vi "stack-temp-tuner.vi"() -> ()   [LabVIEW 2019]
uses:
  <vilib>/Analysis/NI_AALPro.lvlib
panel:
  in  "hyst":sgl=25.0
  in  "boost":sgl=25.0
  in  "boost_delay":u8=25
  in  "Alarm State":bool=TRUE
  in  "Alarm Enable":bool=TRUE
  in  "Mute":bool
  in  "Mute Time (min)":u8=1
  in  "Alarm Diff":u8=30
  in  "Write Manual Coeffs":bool
  in  "Manual Coeffs":sgl[](array[numeric])=[0.0, 1.0]
  in  "Live Data":bool=TRUE
  out "Version":sgl format="%#.1f"
  in  "System Type":u8(ring) items=["Stack Temp", "Auto Draw-Off"]
  in  "pwm_min":u8=25
  in  "ff":sgl
  in  "Output Enable Type":bool
  out "Cal Read 2":sgl format="%#.1g"
  out "Cal Read 1":sgl
  in  "Cal Target 2":sgl=900.0 min=32 max=2000 step=1
  in  "Cal Target 1":sgl=32.0 min=32 max=2000 step=1
  in  "Apply Cal":bool
  out "Temp (deg F)":sgl=78.2392 format="%.1f"
  out "Temp (raw)":sgl=554.0 format="%#.1f"
  in  "Cal Capture 2":bool
  in  "Cal Capture 1":bool
  in  "Received Reset":bool
  out "Parameters Received":bool
  out "Cal Coeffs":sgl[](array[numeric])
  in  "Parameter Request":bool
  in  "Output Enable":bool=TRUE
  in  "pwm_rate":sgl=50.0
  in  "ki":sgl=0.001
  in  "kp":sgl=5.0
  in  "Write Tuning":bool
  in  "Temp Setpoint":sgl=100.0 min=32 max=1832 step=0.1 format="%#.1f"
  out "Live Data":sgl[](array[numeric])=[78.2392, 100.0, 118.0, 9295.232] format="%.1f"
  out "Tuning Chart":T1(graph)={"[0]"=78.2392, "[1]"=100.0, "[2]"=118.0, "[3]"=9295.232, "[4]"=0.0, "[5]"=0.0, "[6]"=0.0, "[7]"=0.0, "[8]"=0.0}
  in  "Stop":bool
  # "Control"
  # "Parameter Request"
  # "Config"
  # "Tuning"
  # "Temp Calibration"
  # "Manual Coeffs"
  # "Stack Temp Alarm"
  # "*Any kp over 5 will cause the command\nstep to increase from 1 to 2.  This is due to\nthe resolution of the temp input (at least\nfor stack temp anyway)"
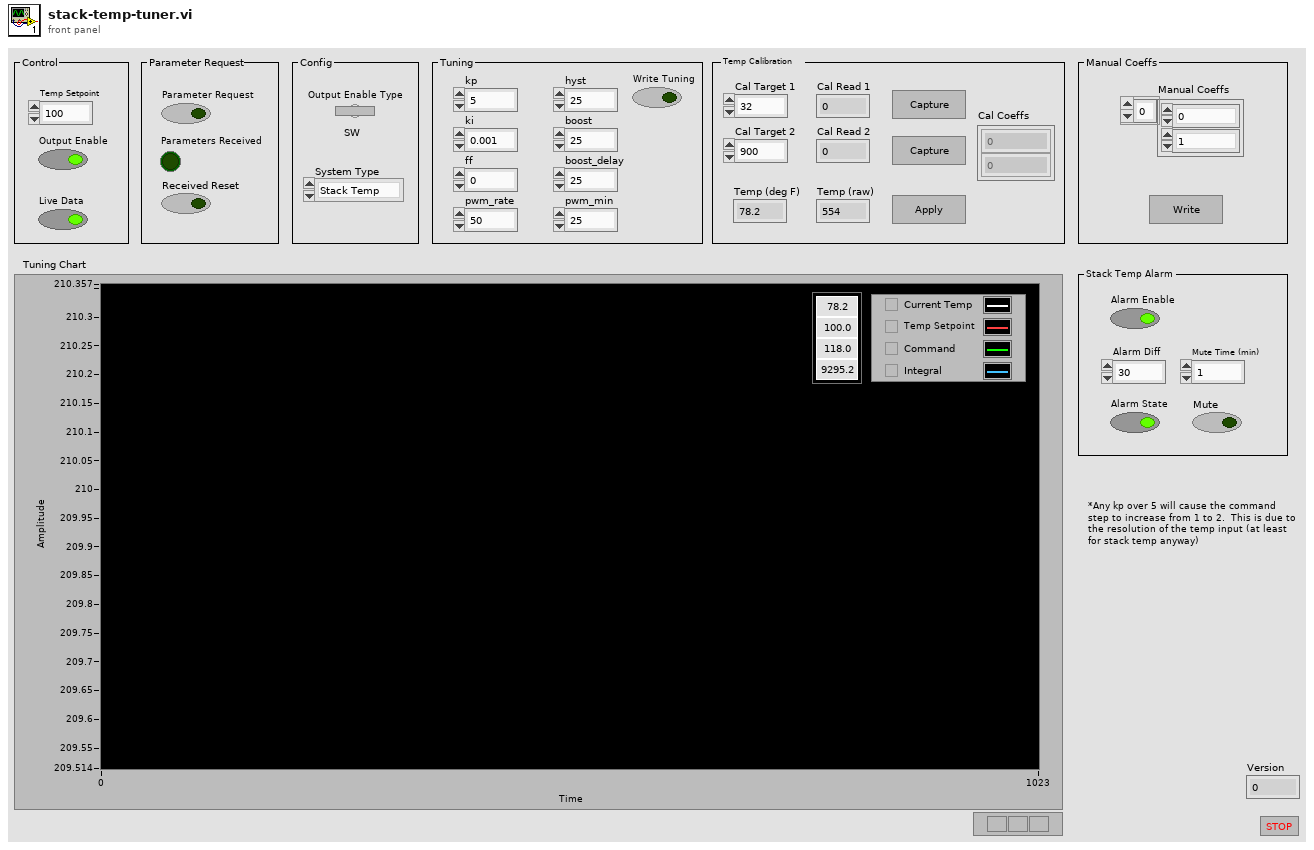
[diagram p1: front panel]
types:
  T1 = cluster{"[0]":sgl, "[1]":sgl, "[2]":sgl, "[3]":sgl, "[4]":sgl, "[5]":sgl, "[6]":sgl, "[7]":sgl, "[8]":sgl}
  T2 = cluster{"Error":errorcluster, "CAN Object":i32, "CAN Msg":u8[], "ArbID":u32, "Cal Coeffs":sgl[], "Current Temp":sgl, "Temp (raw)":sgl, "Temp Setpoint":sgl, "Output Enable":bool, "Parameter Request":bool, "Parameter Received":bool, "Cal Target 1":sgl, "Cal Target 2":sgl, "Cal Read 1":sgl, "Cal Read 2":sgl, "kp":sgl, "ki":sgl, "pwm_rate":sgl, "ff":sgl, "hyst":sgl, "boost":sgl, "pwm_min":u8, "boost_delay":u8, "Temp Setpoint (Live)":sgl, "Integral":sgl, "PWM Command":sgl, "Output Enable Type":bool, "System Type":u8, "Version":sgl, "Alarm Diff":u8, "Alarm Enable":bool, "Mute Time (min)":u8, "Alarm State":bool}
  T3 = enum16{"DEVICE", "HSCAN", "MSCAN", "SWCAN", "LSFTCAN", "FORDSCP", "J1708", "JVPW", "ISO", "FIRE_HSCAN2", "FIRE_MSCAN1", "FIRE_HSCAN3", "FIRE_LIN2", "FIRE_LIN3", "FIRE_LIN4"}
  T4 = cluster{"DeviceType":i32, "Handle":i32, "NumberOfClients":i32, "SerialNumber":i32, "MaxAllowedClients":i32}[]
  T5 = cluster{"DeviceType":i32, "Handle":i32, "NumberOfClients":i32, "SerialNumber":i32, "MaxAllowedClients":i32}
  T6 = typedef "ctl spymessage.ctl" = cluster{"StatusBitField":u32, "StatusBitField2":u32, "TimeHardware":u32, "TimeHardware2":u32, "TimeSystem":u32, "TimeSystem2":u32, "TimeStampHardwareID":u8, "TimeStampHardwareID2":u8, "NetworkID":u8, "NodeID":u8, "Protocol":u8, "MessagePieceID":u8, "ColorID":u8, "NumberBytesHeader":u8, "NumberBytesData":u8, "DescriptionID":u16, "ArbIDOrHeader":u32, "Data [8]":u8[], "AckBytes [8]":u8[], "Value":sgl, "MiscData":u8}
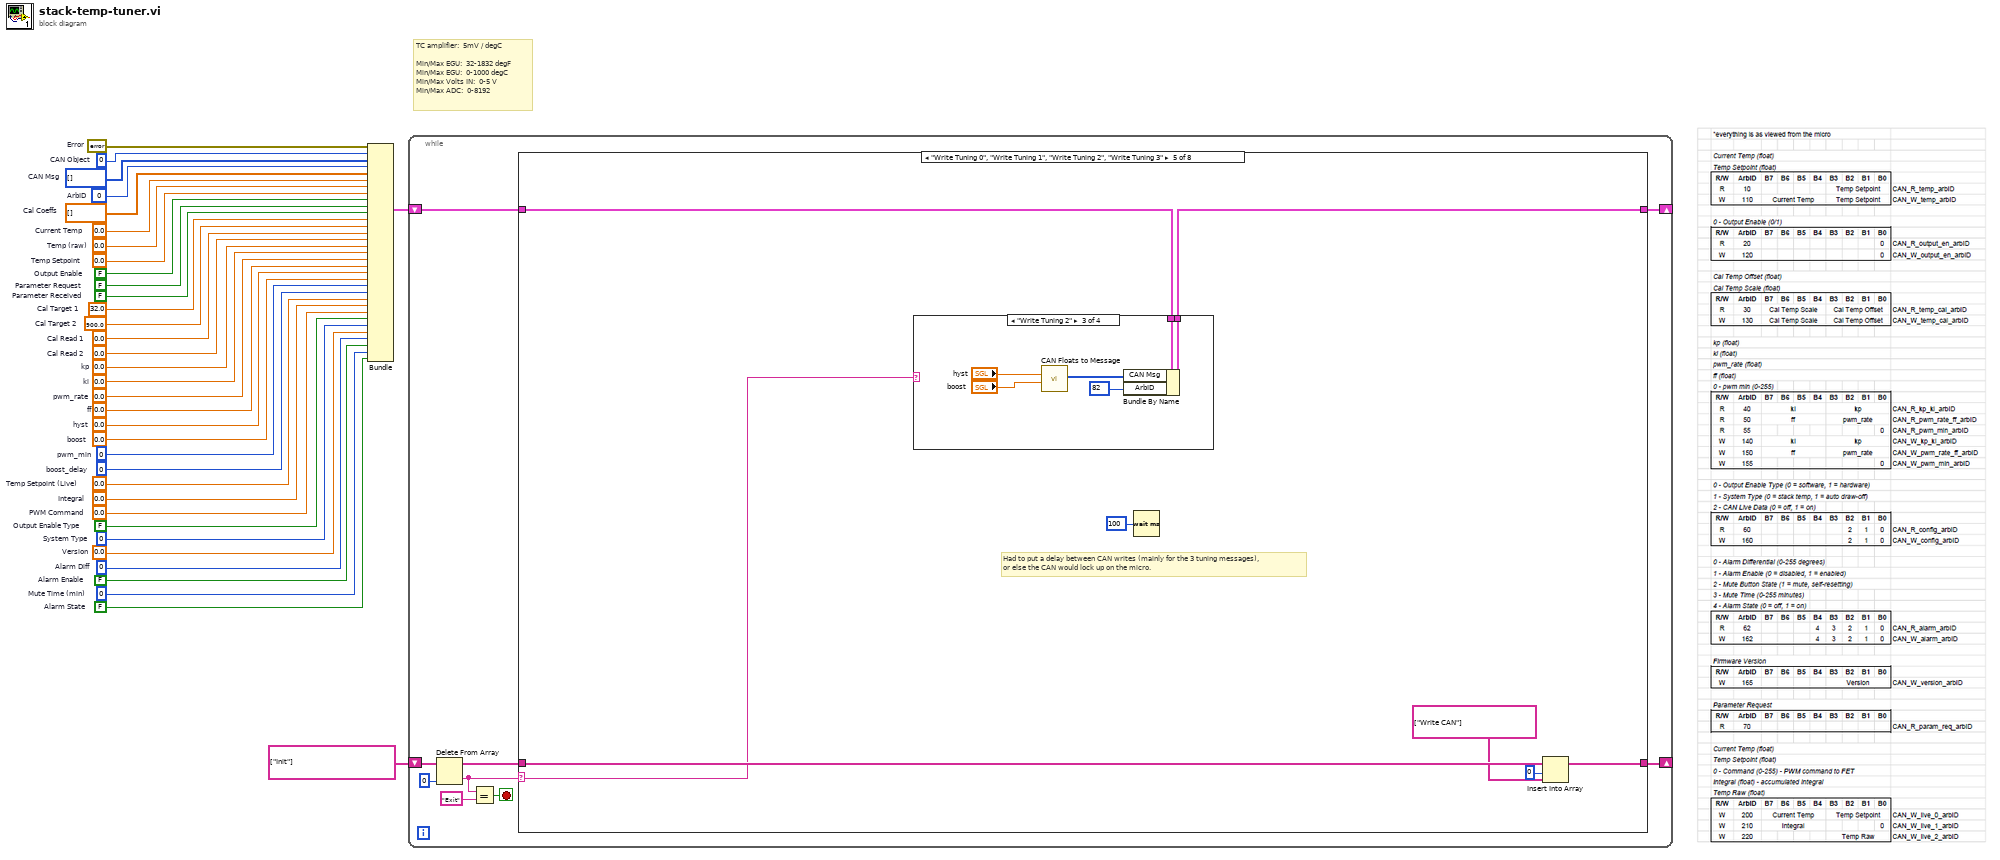
[diagram p0: block diagram]
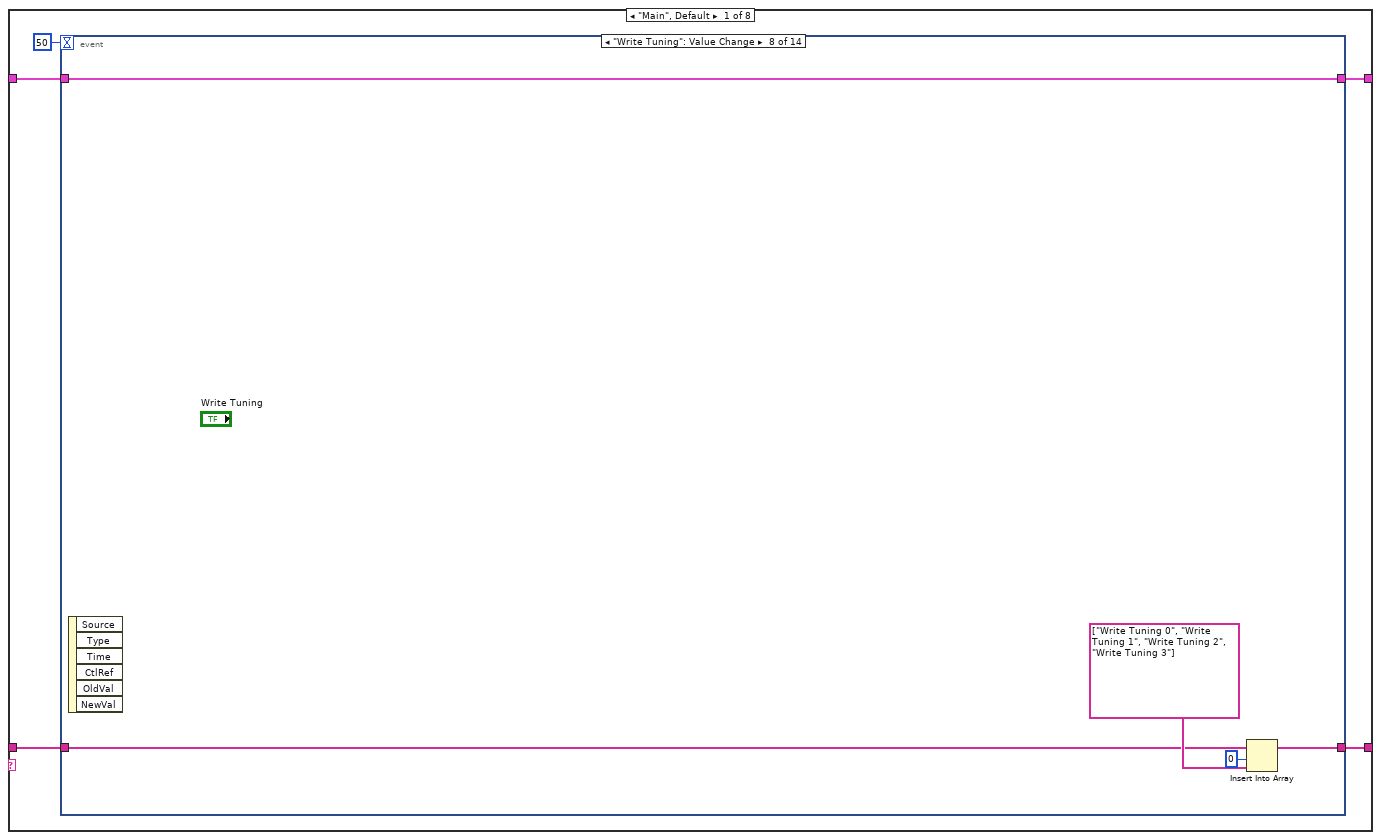
[diagram p2: hidden frame]
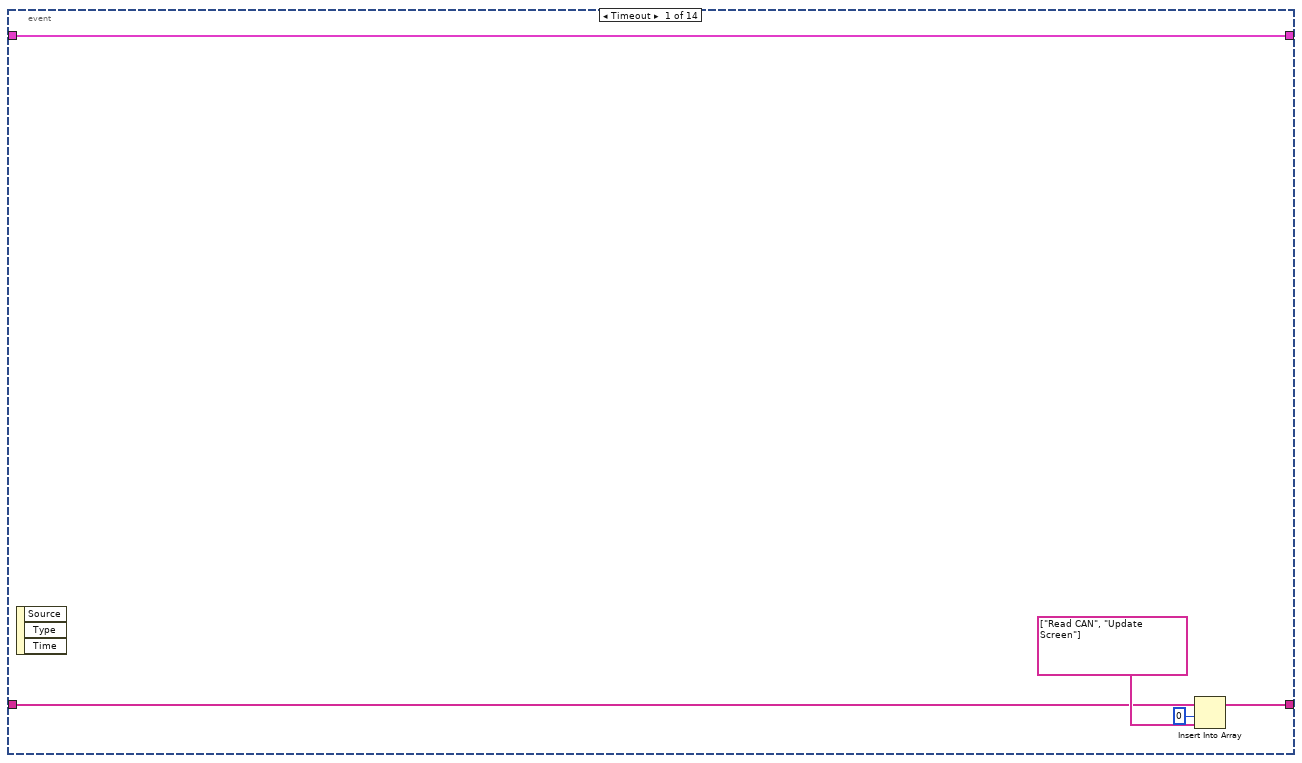
[diagram p3: hidden frame]
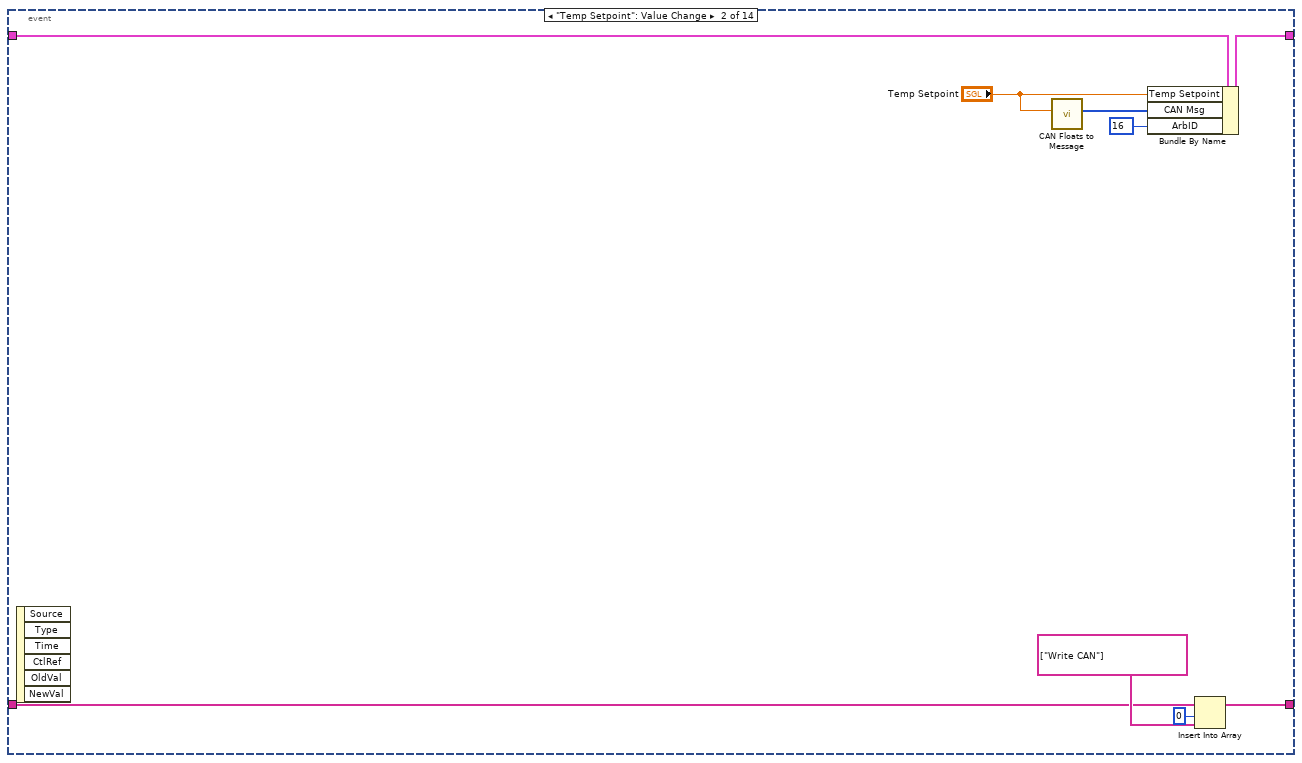
[diagram p4: hidden frame]
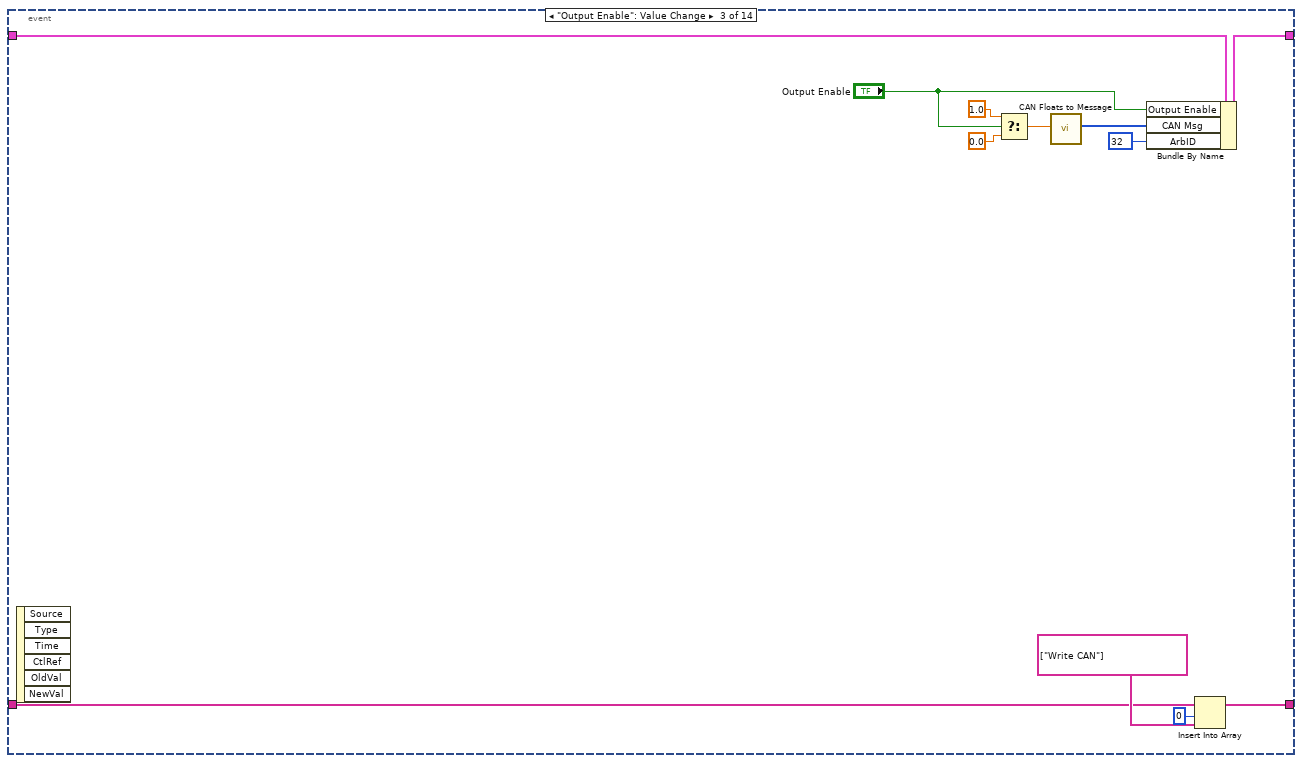
[diagram p5: hidden frame]
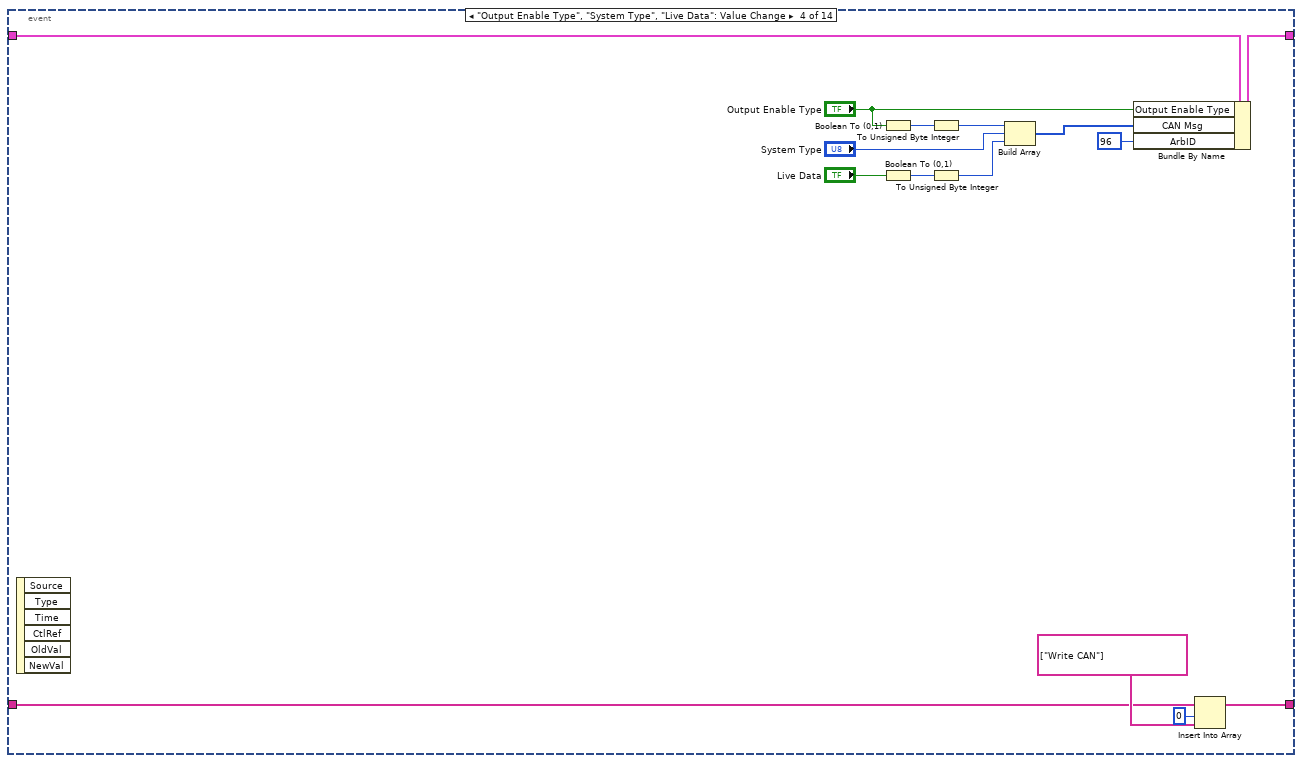
[diagram p6: hidden frame]
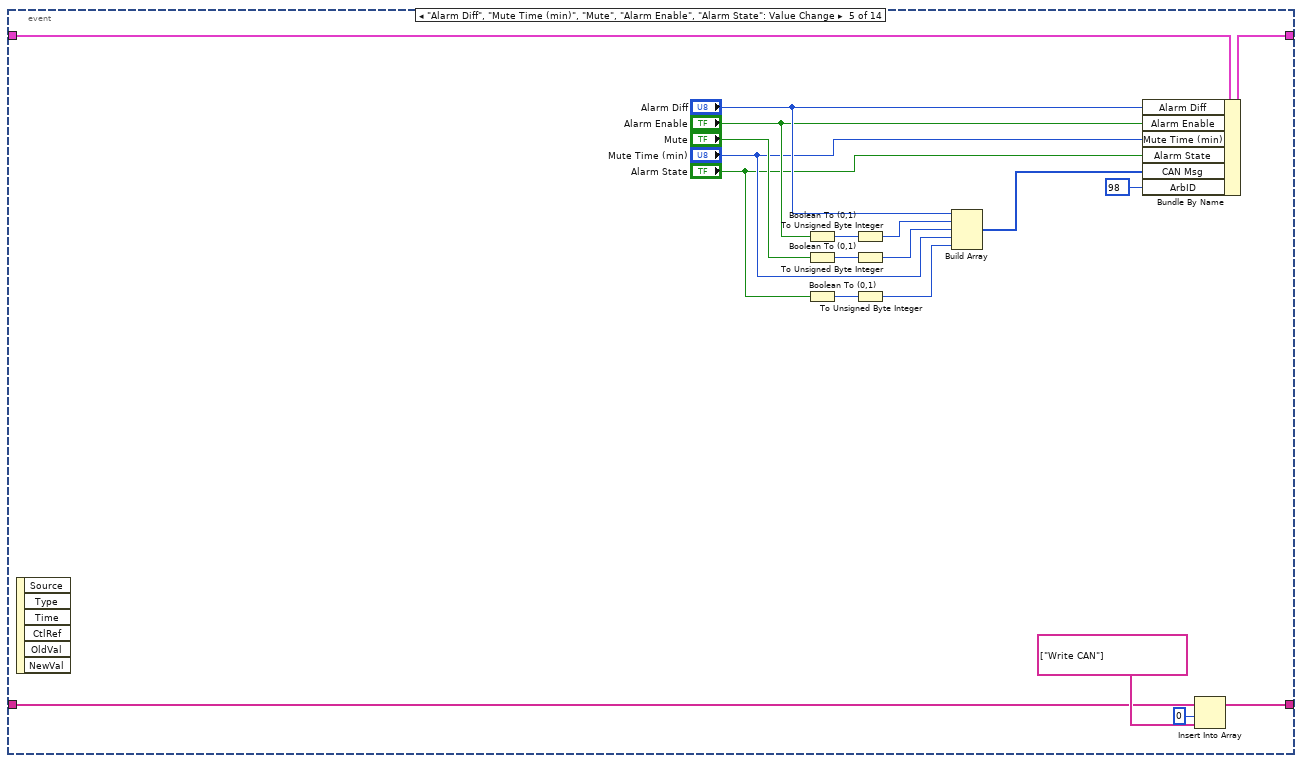
[diagram p7: hidden frame]
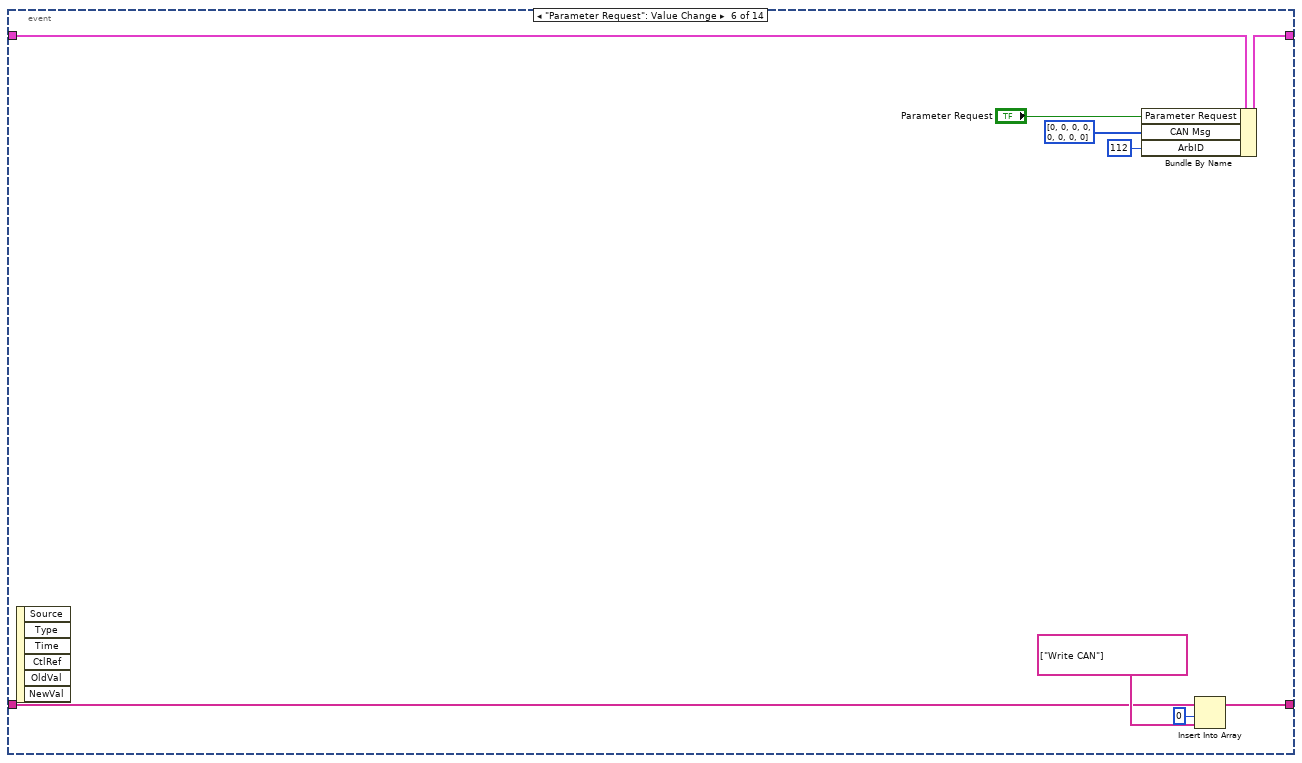
[diagram p8: hidden frame]
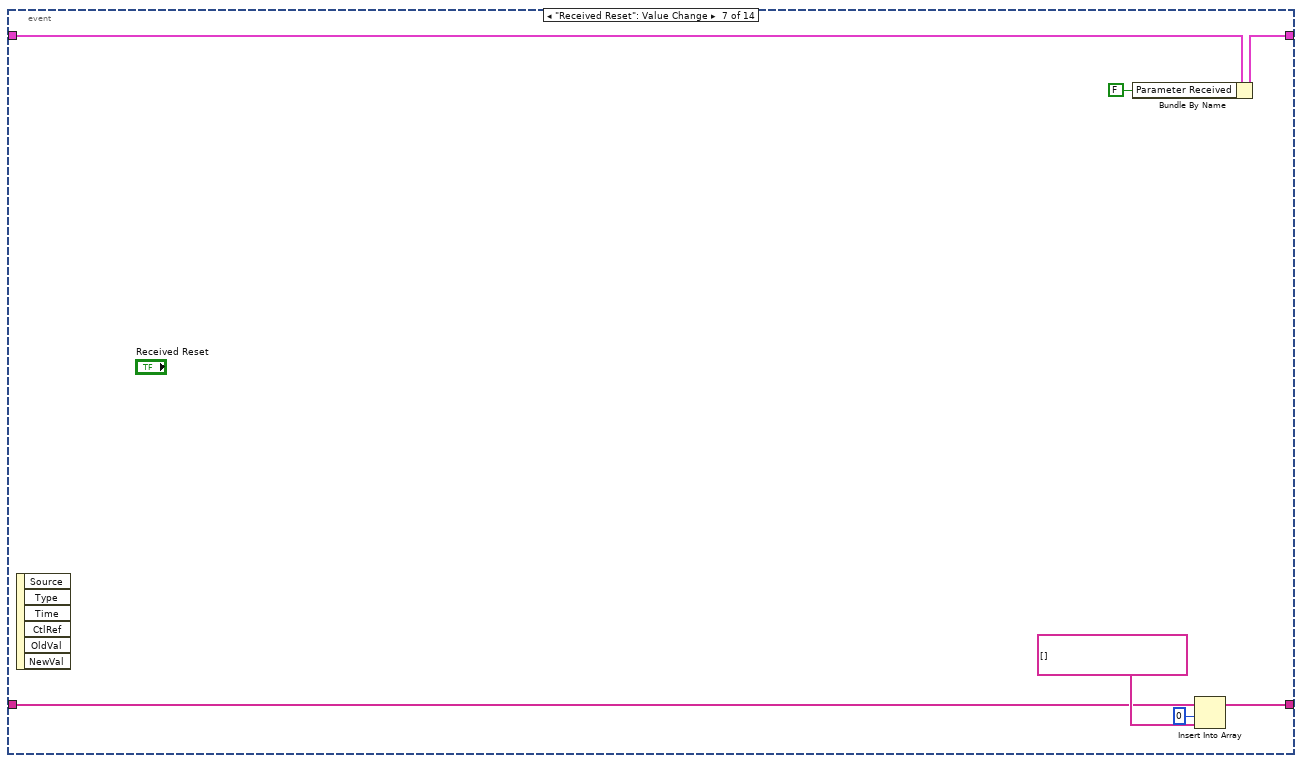
[diagram p9: hidden frame]
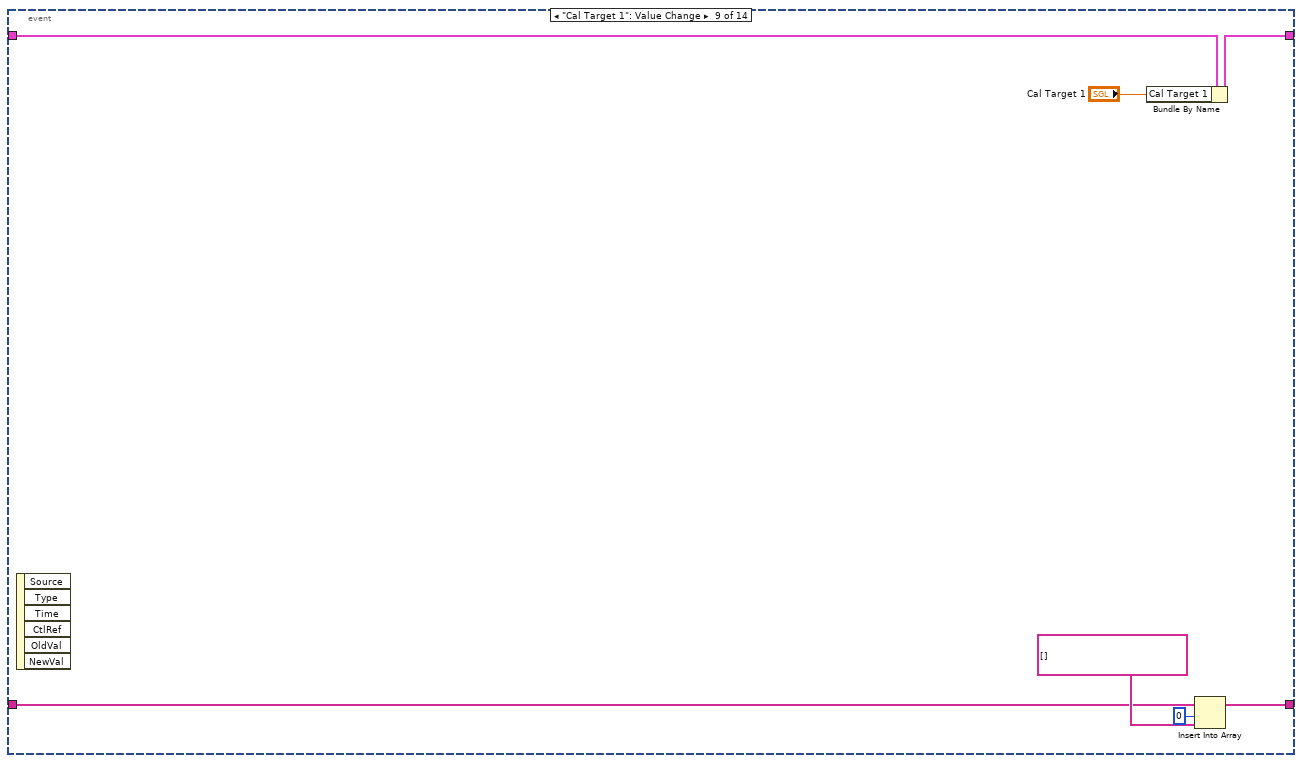
[diagram p10: hidden frame]
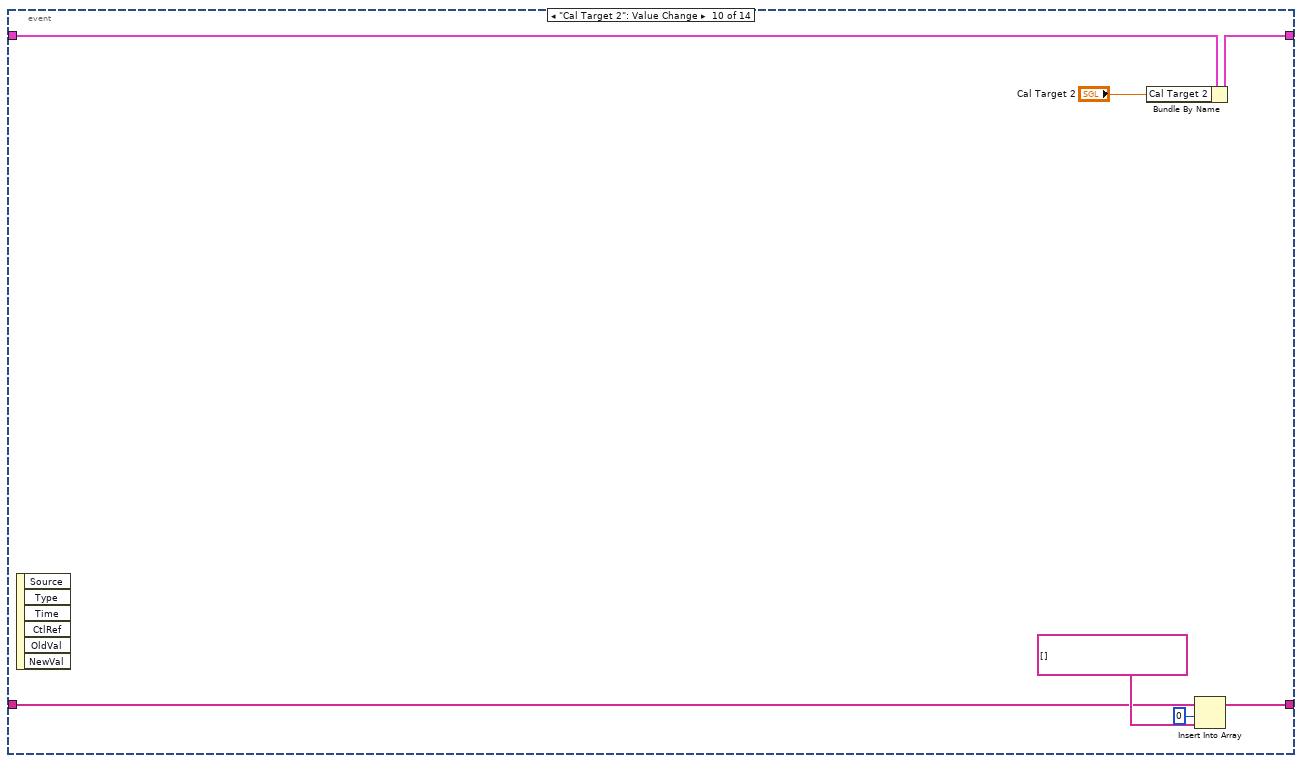
[diagram p11: hidden frame]
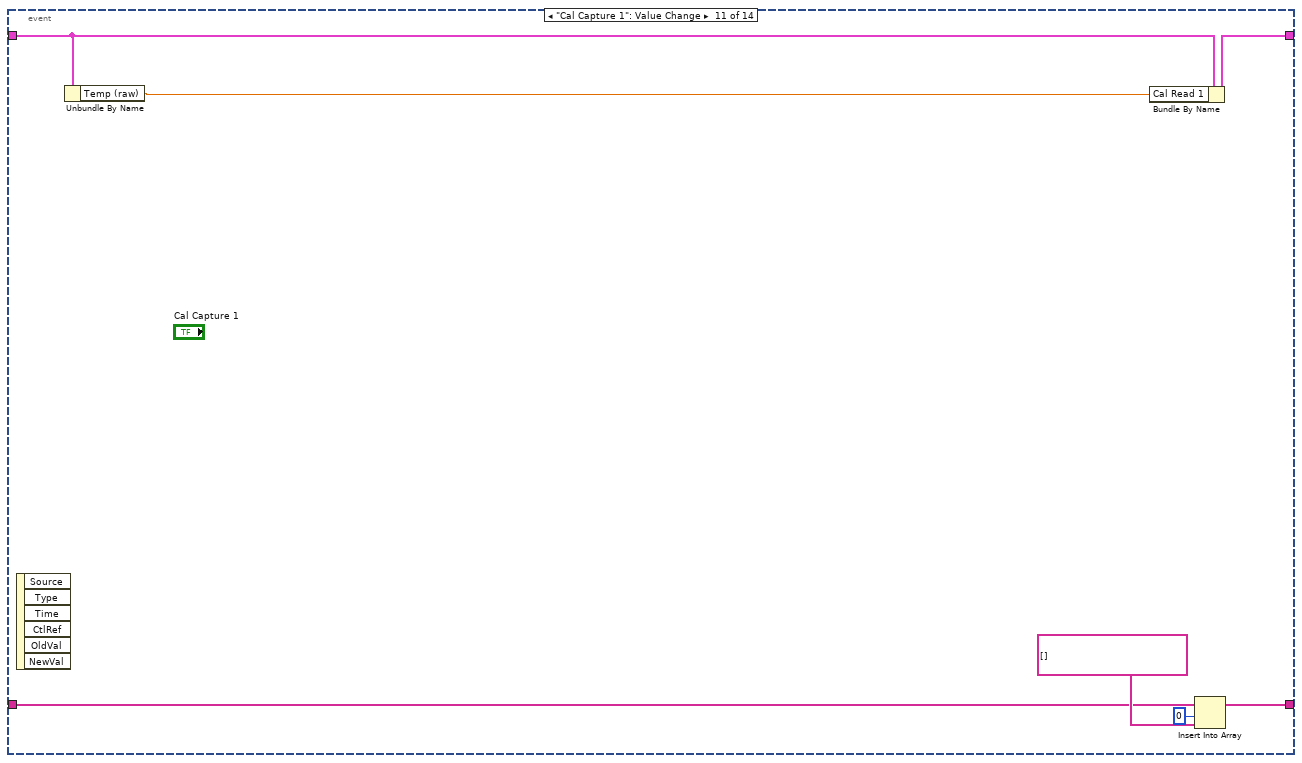
[diagram p12: hidden frame]
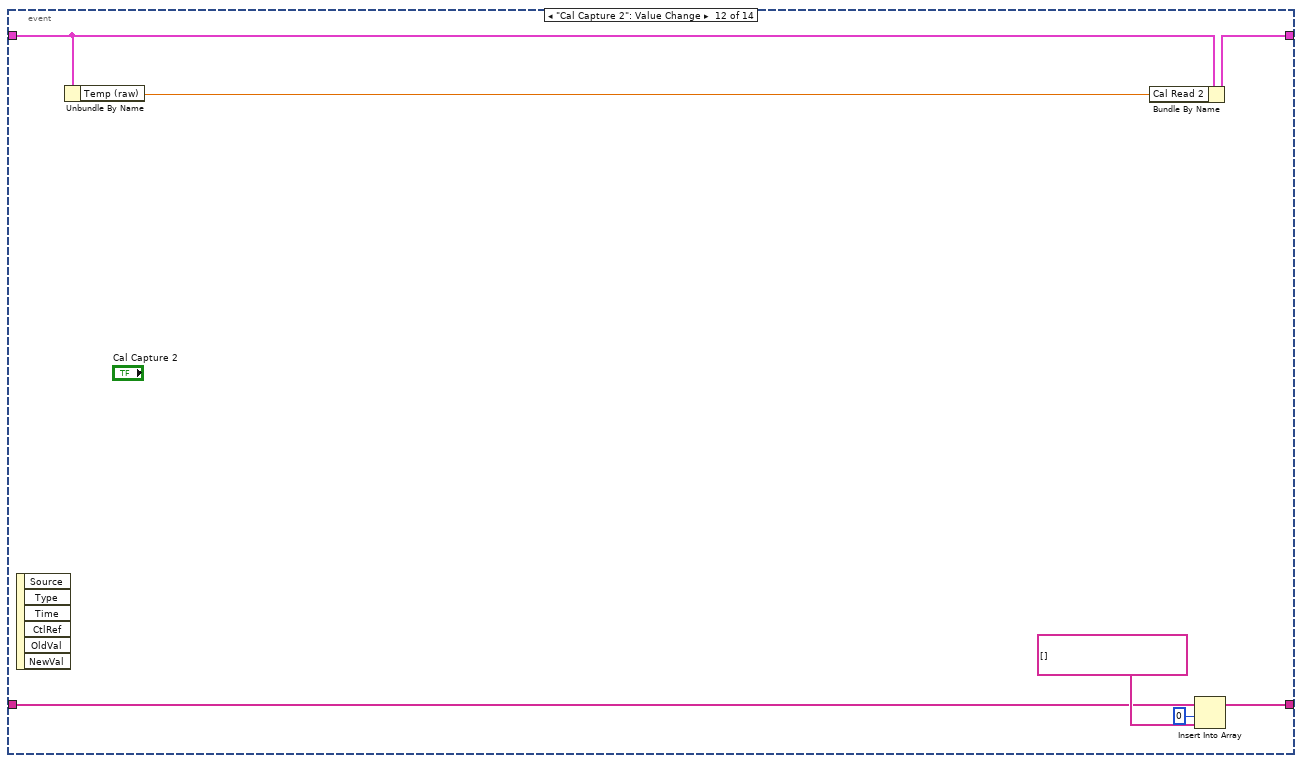
[diagram p13: hidden frame]
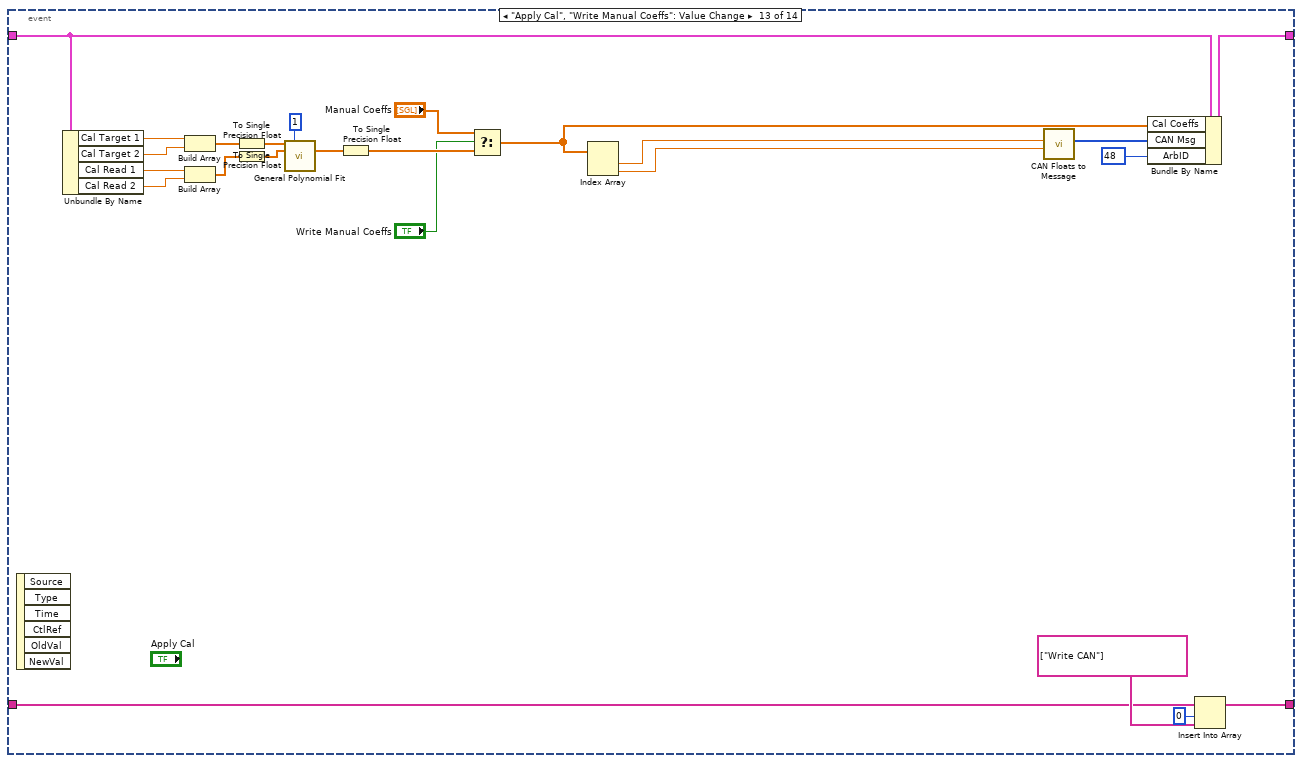
[diagram p14: hidden frame]
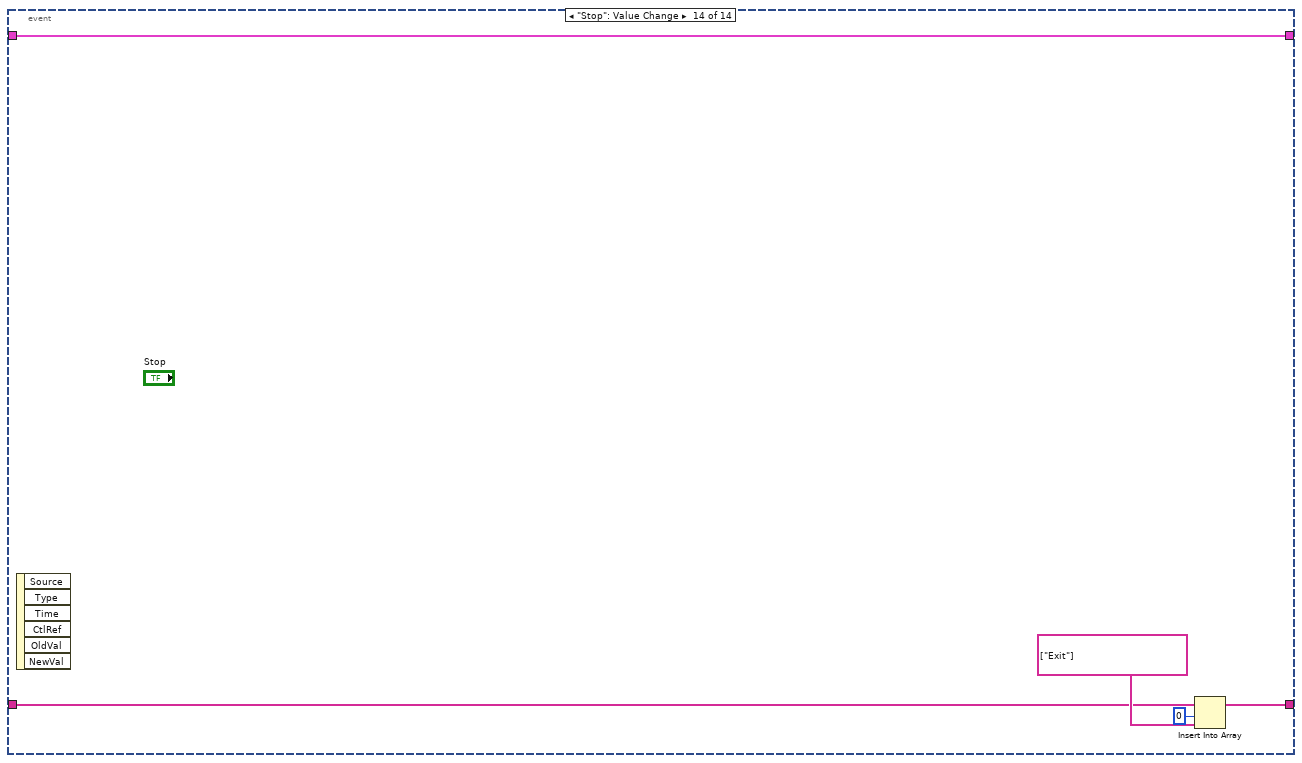
[diagram p15: hidden frame]
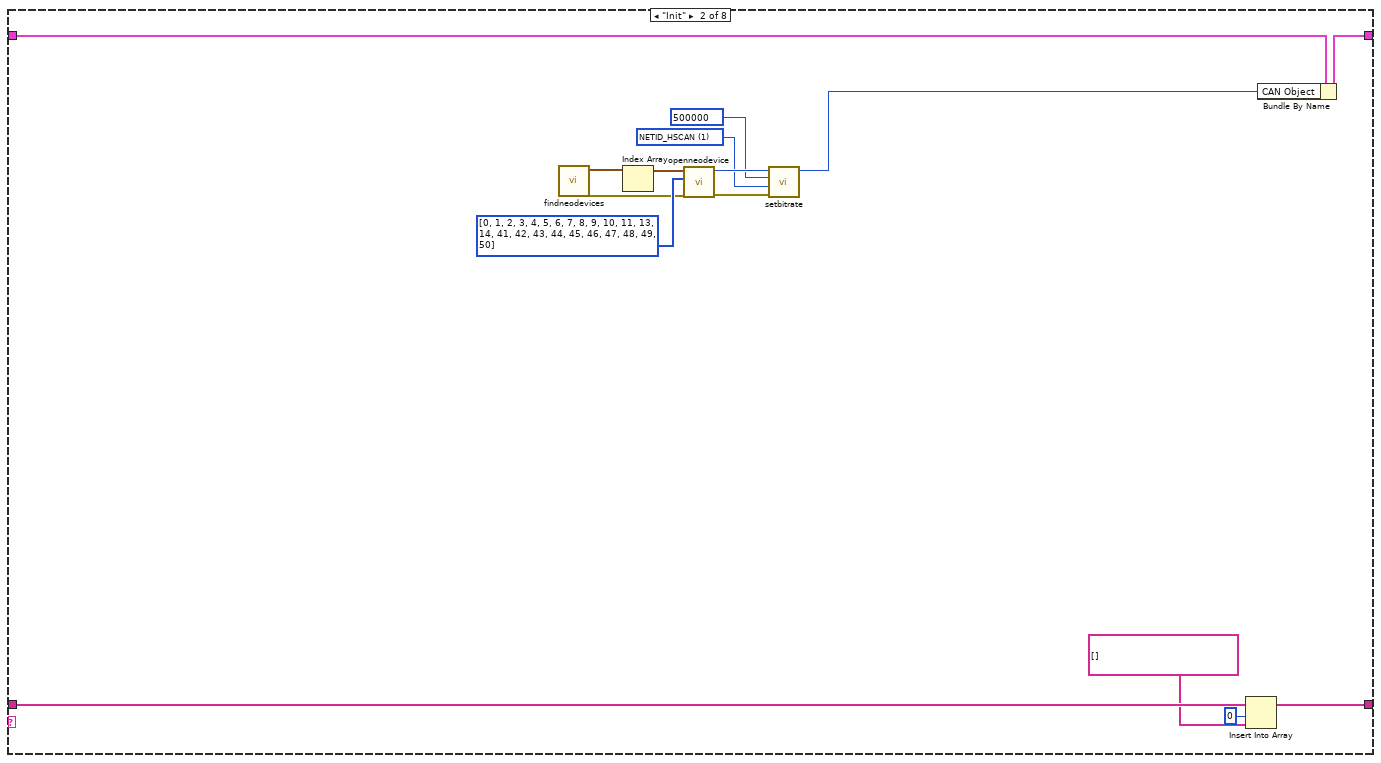
[diagram p16: hidden frame]
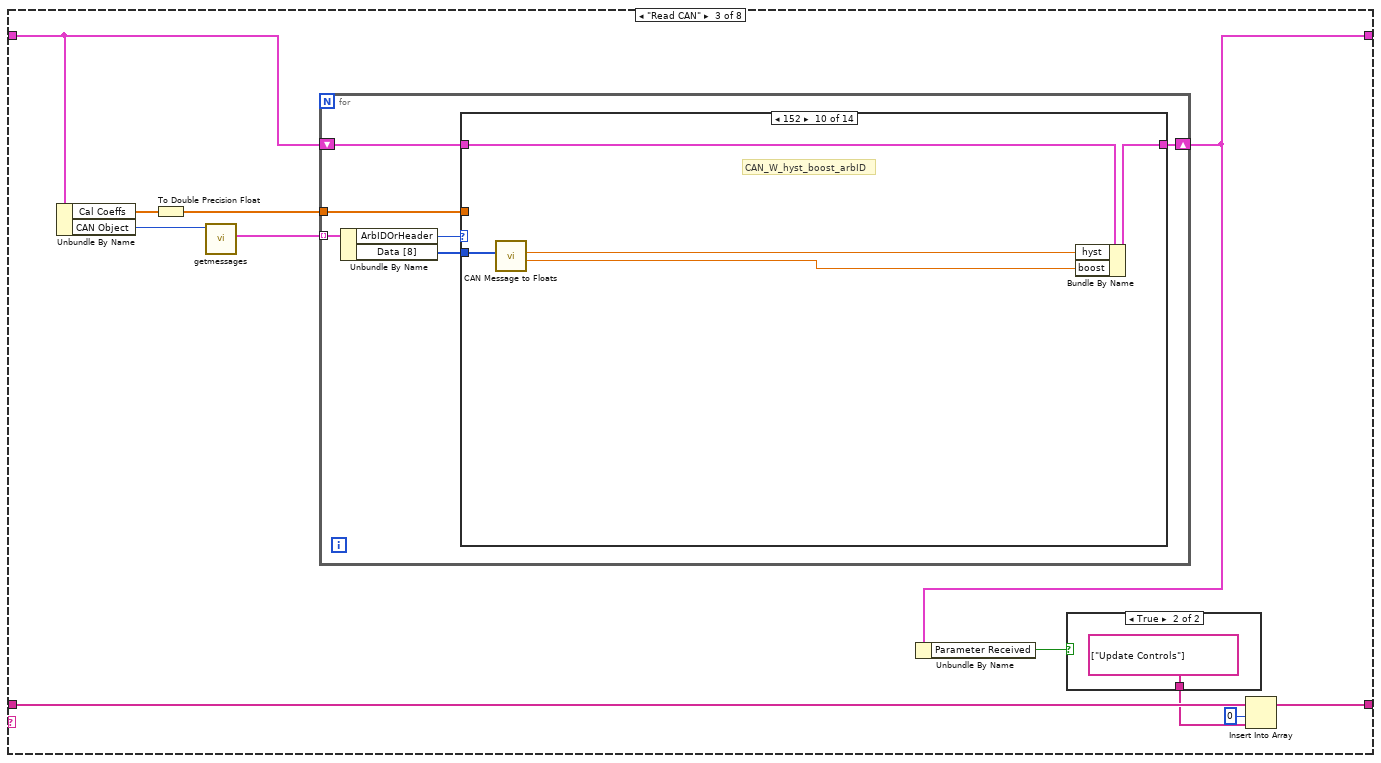
[diagram p17: hidden frame]
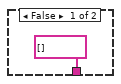
[diagram p18: hidden frame]
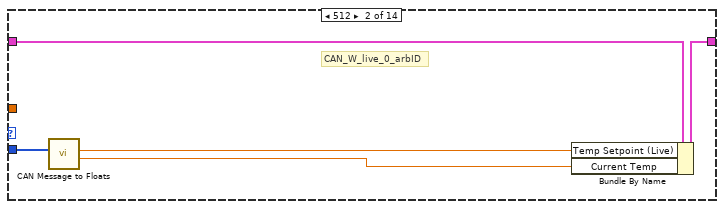
[diagram p20: hidden frame]
diagram:
  w1 = sgl 0.0  # boost
  w2 = sgl 0.0  # hyst
  w3 = u8 0  # boost_delay
  w4 = FALSE  # Alarm State
  w5 = u8 0  # Mute Time (min)
  w6 = FALSE  # Alarm Enable
  w7 = u8 0  # Alarm Diff
  w8 = sgl 0.0  # Version
  w9 = u8 0  # System Type
  w10 = u8 0  # pwm_min
  w11 = sgl 0.0  # ff
  w12 = u32 0  # ArbID
  w13 = u8[] []  # CAN Msg
  w14 = FALSE  # Output Enable Type
  w15 = sgl 0.0  # PWM Command
  w16 = sgl 0.0  # Integral
  w17 = sgl 0.0  # Temp Setpoint (Live)
  w18 = FALSE  # Parameter Received
  w19 = sgl 0.0  # pwm_rate
  w20 = sgl 0.0  # ki
  w21 = sgl 0.0  # kp
  w22 = sgl 0.0  # Temp (raw)
  w23 = sgl 0.0  # Current Temp
  w26 = sgl 900.0  # Cal Target 2
  w27 = sgl 32.0  # Cal Target 1
  w24 = sgl 0.0  # Cal Read 2
  w25 = sgl 0.0  # Cal Read 1
  w28 = FALSE  # Parameter Request
  w29 = FALSE  # Output Enable
  w30 = sgl 0.0  # Temp Setpoint
  w31 = sgl[] []  # Cal Coeffs
  w32 = 0  # CAN Object
  w34 = errorcluster {"status"=FALSE, "code"=0, "source"=""}  # Error
  # "TC amplifier:  5mV / degC\n\nMin/Max EGU:  32-1832 degF\nMin/Max EGU:  0-1000 degC\nMin/Max Volts IN:  0-5 V\nMin/Max ADC:  0-8192"
  n1 = Bundle("Error"=w34, "CAN Object"=w32, "CAN Msg"=w13, "ArbID"=w12, "Cal Coeffs"=w31, "Current Temp"=w23, "Temp (raw)"=w22, "Temp Setpoint"=w30, "Output Enable"=w29, "Parameter Request"=w28, "Parameter Received"=w18, "Cal Target 1"=w27, "Cal Target 2"=w26, "Cal Read 1"=w25, "Cal Read 2"=w24, "kp"=w21, "ki"=w20, "pwm_rate"=w19, "ff"=w11, "hyst"=w2, "boost"=w1, "pwm_min"=w10, "boost_delay"=w3, "Temp Setpoint (Live)"=w17, "Integral"=w16, "PWM Command"=w15, "Output Enable Type"=w14, "System Type"=w9, "Version"=w8, "Alarm Diff"=w7, "Alarm Enable"=w6, "Mute Time (min)"=w5, "Alarm State"=w4) -> (w33:T2)  [unwired: 1 in]
  n2 = while {
    shift-right: [w39] -> _
    shift-left: string[] ["Init"] -> [w44]
    shift-right: [w36] -> _
    shift-left: w33 -> [w37]
    stop <- w40 stop-if-true
    n3 = Delete From Array(array=w44, index=0 ("length")) -> (deleted portion=w41:string, array with subset deleted=w38:string[])  [unwired: 1 in]
    n4 = Equal?(x=w41, y="Exit") -> (x = y?=w40:bool)
    n5 = case shown="\"Write Tuning 0\", \"Write Tuning 1\", \"Write Tuning 2\", \"Write Tuning 3\"" w41 {
      selector: w41 -> [_ _ _ _ w309 _ _ _]
      tunnel: [w45 w191 w213 w307 w315 w357 w377 w383] -> w39
      tunnel: w38 -> [w46 w190 w212 w306 w314 w356 w376 w382]
      tunnel: w37 -> [w49 w193 w206 w299 w310 w345 w365 w379]
      tunnel: [w48 w194 w204 w300 w311 w345 w365 w379] -> w36
      frame "Main", Default {
        n6 = event shown="[7] \"Write Tuning\": Value Change" {
          selector: _ -> [_ _ _ _ _ _ _ _ _ _ _ _ _ _]
          dyn-events: _ -> [_ _ _ _ _ _ _ _ _ _ _ _ _ _]
          timeout: 50 -> [_ _ _ _ _ _ _ _ _ _ _ _ _ _]
          tunnel: w49 -> [w54 w58 w69 w85 w104 w113 w120 w126 w132 w139 w146 w153 w165 w183]
          tunnel: [w54 w59 w68 w84 w103 w112 w121 w126 w133 w140 w147 w154 w176 w183] -> w48
          tunnel: w46 -> [w51 w61 w73 w88 w107 w116 w123 w128 w135 w142 w149 w156 w180 w185]
          tunnel: [w50 w60 w72 w87 w106 w115 w122 w127 w134 w141 w148 w155 w179 w184] -> w45
          event Timeout {
            n7 = event-data() -> ()  [unwired: 1 in, 3 out]
            n8 = Insert Into Array(array=w51, index=0, new element=string[] ["Read CAN", "Update Screen"]) -> (w50:string[])
          }
          event "Temp Setpoint": Value Change {
            n9 = event-data() -> ()  [unwired: 1 in, 6 out]
            n10 = call "CAN Floats to Message.vi"("Float_0"="Temp Setpoint") -> ("CAN Message"=w56:u8[])  [unwired: 10 in]
            n11 = Bundle By Name(cluster=w58, "Temp Setpoint"="Temp Setpoint", "CAN Msg"=w56, "ArbID"=u32 16) -> (w59:T2)
            n12 = Insert Into Array(array=w61, index=0, new element=string[] ["Write CAN"]) -> (w60:string[])
          }
          event "Output Enable": Value Change {
            n13 = event-data() -> ()  [unwired: 1 in, 6 out]
            n14 = Select(t=sgl 1.0, s="Output Enable", f=sgl 0.0) -> (s? t:f=w65:sgl)
            n15 = call "CAN Floats to Message.vi"("Float_0"=w65) -> ("CAN Message"=w71:u8[])  [unwired: 10 in]
            n16 = Bundle By Name(cluster=w69, "Output Enable"="Output Enable", "CAN Msg"=w71, "ArbID"=u32 32) -> (w68:T2)
            n17 = Insert Into Array(array=w73, index=0, new element=string[] ["Write CAN"]) -> (w72:string[])
          }
          event "Output Enable Type", "System Type", "Live Data": Value Change {
            n18 = event-data() -> ()  [unwired: 1 in, 6 out]
            n19 = Boolean To (0,1)(Boolean="Output Enable Type") -> (0, 1=w78:i16)
            n20 = Boolean To (0,1)(Boolean="Live Data") -> (0, 1=w80:i16)
            n21 = To Unsigned Byte Integer(number=w78) -> (unsigned 8bit integer=w77:u8)
            n22 = To Unsigned Byte Integer(number=w80) -> (unsigned 8bit integer=w79:u8)
            n23 = Build Array(w77, "System Type", w79) -> (w82:u8[])
            n24 = Bundle By Name(cluster=w85, "Output Enable Type"="Output Enable Type", "CAN Msg"=w82, "ArbID"=u32 96) -> (w84:T2)
            n25 = Insert Into Array(array=w88, index=0, new element=string[] ["Write CAN"]) -> (w87:string[])
          }
          event "Alarm Diff", "Mute Time (min)", "Mute", "Alarm Enable", "Alarm State": Value Change {
            n26 = event-data() -> ()  [unwired: 1 in, 6 out]
            n27 = Boolean To (0,1)(Boolean="Alarm Enable") -> (0, 1=w102:i16)
            n28 = Boolean To (0,1)(Boolean="Mute") -> (0, 1=w100:i16)
            n29 = Boolean To (0,1)(Boolean="Alarm State") -> (0, 1=w99:i16)
            n30 = To Unsigned Byte Integer(number=w102) -> (unsigned 8bit integer=w97:u8)
            n31 = To Unsigned Byte Integer(number=w100) -> (unsigned 8bit integer=w95:u8)
            n32 = To Unsigned Byte Integer(number=w99) -> (unsigned 8bit integer=w92:u8)
            n33 = Build Array("Alarm Diff", w97, w95, "Mute Time (min)", w92) -> (w91:u8[])
            n34 = Bundle By Name(cluster=w104, "Alarm Diff"="Alarm Diff", "Alarm Enable"="Alarm Enable", "Mute Time (min)"="Mute Time (min)", "Alarm State"="Alarm State", "CAN Msg"=w91, "ArbID"=u32 98) -> (w103:T2)
            n35 = Insert Into Array(array=w107, index=0, new element=string[] ["Write CAN"]) -> (w106:string[])
          }
          event "Parameter Request": Value Change {
            n36 = event-data() -> ()  [unwired: 1 in, 6 out]
            n37 = Bundle By Name(cluster=w113, "Parameter Request"="Parameter Request", "CAN Msg"=u8[] [0, 0, 0, 0, 0, 0, 0, 0], "ArbID"=u32 112) -> (w112:T2)
            n38 = Insert Into Array(array=w116, index=0, new element=string[] ["Write CAN"]) -> (w115:string[])
          }
          event "Received Reset": Value Change {
            n39 = event-data() -> ()  [unwired: 1 in, 6 out]
            n40 = Bundle By Name(cluster=w120, "Parameter Received"=FALSE) -> (w121:T2)
            n41 = Insert Into Array(array=w123, index=0, new element=string[] []) -> (w122:string[])
          }
          event "Write Tuning": Value Change {
            n42 = event-data() -> ()  [unwired: 1 in, 6 out]
            n43 = Insert Into Array(array=w128, index=0, new element=string[] ["Write Tuning 0", "Write Tuning 1", "Write Tuning 2", "Write Tuning 3"]) -> (w127:string[])
          }
          event "Cal Target 1": Value Change {
            n44 = event-data() -> ()  [unwired: 1 in, 6 out]
            n45 = Bundle By Name(cluster=w132, "Cal Target 1"="Cal Target 1") -> (w133:T2)
            n46 = Insert Into Array(array=w135, index=0, new element=string[] []) -> (w134:string[])
          }
          event "Cal Target 2": Value Change {
            n47 = event-data() -> ()  [unwired: 1 in, 6 out]
            n48 = Bundle By Name(cluster=w139, "Cal Target 2"="Cal Target 2") -> (w140:T2)
            n49 = Insert Into Array(array=w142, index=0, new element=string[] []) -> (w141:string[])
          }
          event "Cal Capture 1": Value Change {
            n50 = event-data() -> ()  [unwired: 1 in, 6 out]
            n51 = Unbundle By Name(w146) -> ("Temp (raw)"=w145:sgl)
            n52 = Bundle By Name(cluster=w146, "Cal Read 1"=w145) -> (w147:T2)
            n53 = Insert Into Array(array=w149, index=0, new element=string[] []) -> (w148:string[])
          }
          event "Cal Capture 2": Value Change {
            n54 = event-data() -> ()  [unwired: 1 in, 6 out]
            n55 = Unbundle By Name(w153) -> ("Temp (raw)"=w152:sgl)
            n56 = Bundle By Name(cluster=w153, "Cal Read 2"=w152) -> (w154:T2)
            n57 = Insert Into Array(array=w156, index=0, new element=string[] []) -> (w155:string[])
          }
          event "Apply Cal", "Write Manual Coeffs": Value Change {
            n58 = event-data() -> ()  [unwired: 1 in, 6 out]
            n59 = Unbundle By Name(w165) -> ("Cal Target 1"=w175:sgl, "Cal Target 2"=w174:sgl, "Cal Read 1"=w173:sgl, "Cal Read 2"=w172:sgl)
            n60 = Build Array(w175, w174) -> (w171:sgl[])
            n61 = Build Array(w173, w172) -> (w168:sgl[])
            n62 = To Single Precision Float(number=w171) -> (single precision float=w169:sgl[])
            n63 = To Single Precision Float(number=w168) -> (single precision float=w167:sgl[])
            n64 = call <vilib>:"General Polynomial Fit.vi"("Y"=w169, "polynomial order"=1, "X"=w167) -> ("Polynomial Coefficients"=w170:dbl[])  [unwired: 9 in, 3 out]
            n65 = To Single Precision Float(number=w170) -> (single precision float=w162:sgl[])
            n66 = Select(t="Manual Coeffs", s="Write Manual Coeffs", f=w162) -> (s? t:f=w161:sgl[])
            n67 = Index Array(array=w161) -> (element #1=w164:sgl, element #2=w163:sgl)  [unwired: 2 in]
            n68 = call "CAN Floats to Message.vi"("Float_1"=w163, "Float_0"=w164) -> ("CAN Message"=w178:u8[])  [unwired: 9 in]
            n69 = Bundle By Name(cluster=w165, "Cal Coeffs"=w161, "CAN Msg"=w178, "ArbID"=u32 48) -> (w176:T2)
            n70 = Insert Into Array(array=w180, index=0, new element=string[] ["Write CAN"]) -> (w179:string[])
          }
          event "Stop": Value Change {
            n71 = event-data() -> ()  [unwired: 1 in, 6 out]
            n72 = Insert Into Array(array=w185, index=0, new element=string[] ["Exit"]) -> (w184:string[])
          }
        }
      }
      frame "Init" {
        w200 = i8 1 items=["NETID_DEVICE"=0, "NETID_HSCAN"=1, "NETID_MSCAN"=2, "NETID_SWCAN"=3, "NETID_LSFTCAN"=4, "NETID_FORDSCP"=5, "NETID_J1708"=6, "NETID_AUX"=7, "NETID_JVPW"=8, "NETID_ISO_LIN"=9, "NETID_ISOPIC"=10, "NETID_MAIN51"=11, "NETID_SCI"=13, "NETID_ISO2"=14, "NETID_FIRE_HSCAN1"=41, "NETID_FIRE_HSCAN2"=42, "NETID_FIRE_MSCAN1"=43, "NETID_FIRE_MSCAN2_HSCAN3"=44, "NETID_FIRE_SWCAN"=45, "NETID_FIRE_LSFT"=46, "NETID_FIRE_LIN1"=47, "NETID_FIRE_LIN2"=48, "NETID_FIRE_LIN3"=49, "NETID_FIRE_LIN4"=50] ("NetworkID")
        w199 = 500000 items=["20000"=20000, "33333"=33333, "50000"=50000, "62500"=62500, "83333"=83333, "100000"=100000, "125000"=125000, "250000"=250000, "500000"=500000, "800000"=800000, "1000000"=1000000] ("Bit Rate")
        w198 = i8[] [0, 1, 2, 3, 4, 5, 6, 7, 8, 9, 10, 11, 13, 14, 41, 42, 43, 44, 45, 46, 47, 48, 49, 50] items=["NETID_DEVICE"=0, "NETID_HSCAN"=1, "NETID_MSCAN"=2, "NETID_SWCAN"=3, "NETID_LSFTCAN"=4, "NETID_FORDSCP"=5, "NETID_J1708"=6, "NETID_AUX"=7, "NETID_JVPW"=8, "NETID_ISO_LIN"=9, "NETID_ISOPIC"=10, "NETID_MAIN51"=11, "NETID_SCI"=13, "NETID_ISO2"=14, "NETID_FIRE_HSCAN1"=41, "NETID_FIRE_HSCAN2"=42, "NETID_FIRE_MSCAN1"=43, "NETID_FIRE_MSCAN2_HSCAN3"=44, "NETID_FIRE_SWCAN"=45, "NETID_FIRE_LSFT"=46, "NETID_FIRE_LIN1"=47, "NETID_FIRE_LIN2"=48, "NETID_FIRE_LIN3"=49, "NETID_FIRE_LIN4"=50] ("bNetworkIDs")
        n73 = call "findneodevices.vi"() -> ("error out"=w196:errorcluster, "NeoDevices {}"=w195:T4)  [unwired: 3 in, 7 out]
        n74 = Index Array(array=w195) -> (element=w197:T5)  [unwired: 1 in]
        n75 = call "openneodevice.vi"("error in (no error)"=w196, "bNetworkIDs"=w198, "NeoDevice{}"=w197) -> ("error out"=w202:errorcluster, "hObject"=w201:i32)  [unwired: 2 in, 5 out]
        n76 = call "setbitrate.vi"("error in (no error)"=w202, "NetworkID"=w200, "BitRate"=w199, "hObject"=w201) -> ("hObject Out"=w192:i32)  [unwired: 7 out]
        n77 = Insert Into Array(array=w190, index=0, new element=string[] []) -> (w191:string[])
        n78 = Bundle By Name(cluster=w193, "CAN Object"=w192) -> (w194:T2)
      }
      frame "Read CAN" {
        n79 = Unbundle By Name(w206) -> ("Cal Coeffs"=w207:sgl[], "CAN Object"=w209:i32)
        n80 = To Double Precision Float(number=w207) -> (double precision float=w205:dbl[])
        n81 = call "getmessages.vi"("hObject"=w209) -> ("pMsgs"=w208:T6[])  [unwired: 1 in, 9 out]
        n82 = for {
          tunnel: w208 -> [w221] mode=indexing
          tunnel: w205 -> [w220]
          shift-right: [w217] -> w204
          shift-left: w206 -> [w218]
          n83 = Unbundle By Name(w221) -> ("ArbIDOrHeader"=w219:u32, "Data [8]"=w216:u8[])
          n84 = case shown="152" w219 {
            tunnel: w220 -> [_ _ _ _ _ _ _ _ _ _ _ _ _ _]
            tunnel: w218 -> [w222 w227 w232 w236 w241 w246 w252 w257 w262 w267 w272 w278 w287 w291]
            tunnel: [w222 w226 w231 w235 w242 w247 w253 w258 w263 w268 w273 w279 w288 w292] -> w217
            tunnel: w216 -> [_ w225 w230 w234 w239 w245 w251 w256 w261 w266 w271 w276 w286 w290]
            frame Default {
              # "No CAN messages available."
            }
            frame 512 {
              # "CAN_W_live_0_arbID"
              n85 = call "CAN Message to Floats.vi"("CAN Message"=w225) -> ("Float_1"=w223:sgl, "Float_0"=w224:sgl)  [unwired: 9 in]
              n86 = Bundle By Name(cluster=w227, "Temp Setpoint (Live)"=w224, "Current Temp"=w223) -> (w226:T2)
            }
            frame 528 {
              # "CAN_W_live_1_arbID"
              n87 = call "CAN Message to Floats.vi"("CAN Message"=w230) -> ("Float_1"=w228:sgl, "Float_0"=w229:sgl)  [unwired: 9 in]
              n88 = Bundle By Name(cluster=w232, "PWM Command"=w229, "Integral"=w228) -> (w231:T2)
            }
            frame 544 {
              # "CAN_W_live_2_arbID"
              n89 = call "CAN Message to Floats.vi"("CAN Message"=w234) -> ("Float_0"=w233:sgl)  [unwired: 9 in, 1 out]
              n90 = Bundle By Name(cluster=w236, "Temp (raw)"=w233) -> (w235:T2)
            }
            frame 272 {
              # "CAN_W_temp_arbID"
              n91 = call "CAN Message to Floats.vi"("CAN Message"=w239) -> ("Float_1"=w237:sgl, "Float_0"=w238:sgl)  [unwired: 9 in]
              n92 = Bundle By Name(cluster=w241, "Temp Setpoint"=w238, "Current Temp"=w237, "Parameter Received"=TRUE) -> (w242:T2)
            }
            frame 288 {
              # "CAN_W_output_en_arbID"
              n93 = call "CAN Message to Floats.vi"("CAN Message"=w245) -> ("Float_0"=w244:sgl)  [unwired: 9 in, 1 out]
              n94 = Greater Than 0?(x=w244) -> (x > 0?=w243:bool)
              n95 = Bundle By Name(cluster=w246, "Output Enable"=w243) -> (w247:T2)
            }
            frame 304 {
              # "CAN_W_temp_cal_arbID"
              n96 = call "CAN Message to Floats.vi"("CAN Message"=w251) -> ("Float_1"=w249:sgl, "Float_0"=w250:sgl)  [unwired: 9 in]
              n97 = Build Array(w250, w249) -> (w248:sgl[])
              n98 = Bundle By Name(cluster=w252, "Cal Coeffs"=w248) -> (w253:T2)
            }
            frame 320 {
              # "CAN_W_kp_ki_arbID"
              n99 = call "CAN Message to Floats.vi"("CAN Message"=w256) -> ("Float_1"=w254:sgl, "Float_0"=w255:sgl)  [unwired: 9 in]
              n100 = Bundle By Name(cluster=w257, "kp"=w255, "ki"=w254) -> (w258:T2)
            }
            frame 336 {
              # "CAN_W_pwm_rate_ff_arbID"
              n101 = call "CAN Message to Floats.vi"("CAN Message"=w261) -> ("Float_1"=w259:sgl, "Float_0"=w260:sgl)  [unwired: 9 in]
              n102 = Bundle By Name(cluster=w262, "pwm_rate"=w260, "ff"=w259) -> (w263:T2)
            }
            frame 338 {
              # "CAN_W_hyst_boost_arbID"
              n103 = call "CAN Message to Floats.vi"("CAN Message"=w266) -> ("Float_1"=w264:sgl, "Float_0"=w265:sgl)  [unwired: 9 in]
              n104 = Bundle By Name(cluster=w267, "hyst"=w265, "boost"=w264) -> (w268:T2)
            }
            frame 341 {
              # "CAN_W_pwm_min_arbID"
              n105 = Index Array(array=w271) -> (element #1=w270:u8, element #2=w269:u8)  [unwired: 2 in]
              n106 = Bundle By Name(cluster=w272, "pwm_min"=w270, "boost_delay"=w269) -> (w273:T2)
            }
            frame 352 {
              # "CAN_W_config_arbID"
              n107 = Index Array(array=w276) -> (element #1=w275:u8, element #2=w274:u8)  [unwired: 2 in]
              n108 = Greater Than 0?(x=w275) -> (x > 0?=w277:bool)
              n109 = Bundle By Name(cluster=w278, "Output Enable Type"=w277, "System Type"=w274) -> (w279:T2)
            }
            frame 354 {
              # "CAN_W_alarm_arbID"
              n110 = Index Array(array=w286) -> (element #1=w285:u8, element #2=w284:u8, element #4=w282:u8, element #5=w281:u8)  [unwired: 5 in, 1 out]
              n111 = Greater Than 0?(x=w284) -> (x > 0?=w283:bool)
              n112 = Greater Than 0?(x=w281) -> (x > 0?=w280:bool)
              n113 = Bundle By Name(cluster=w287, "Alarm Diff"=w285, "Alarm Enable"=w283, "Mute Time (min)"=w282, "Alarm State"=w280) -> (w288:T2)
            }
            frame 357 {
              # "CAN_W_version_arbID"
              n114 = call "CAN Message to Floats.vi"("CAN Message"=w290) -> ("Float_0"=w289:sgl)  [unwired: 9 in, 1 out]
              n115 = Bundle By Name(cluster=w291, "Version"=w289) -> (w292:T2)
            }
          }
        }
        n116 = Unbundle By Name(w204) -> ("Parameter Received"=w203:bool)
        n117 = case shown="True" w203 {
          tunnel: [string[] [] string[] ["Update Controls"]] -> w211
          frame False {
          }
          frame True {
          }
        }
        n118 = Insert Into Array(array=w212, index=0, new element=w211) -> (w213:string[])
      }
      frame "Write CAN" {
        w301 = 8 items=["0", "1", "2", "3", "4", "5", "6", "7", "8", "9", "10", "11"] ("Number of \nData Bytes")
        n119 = Unbundle By Name(w299) -> ("ArbID"=w297:u32, "CAN Msg"=w296:u8[], "CAN Object"=w294:i32)
        n120 = Reshape Array(w296, 8 ("dimension size")) -> (w295:u8[])
        n121 = call "transmit messages.vi"("extended ID?"=FALSE ("Send Extended ID"), "Network"=T3."HSCAN", "Arb ID"=w297, "Number of \nData Bytes"=w301, "hObject In"=w294, "Data"=w295) -> ()  [unwired: 1 in, 5 out]
        n122 = Bundle By Name(cluster=w299, "Parameter Request"=FALSE) -> (w300:T2)
        n123 = Insert Into Array(array=w306, index=0, new element=string[] []) -> (w307:string[])
      }
      frame "Write Tuning 0", "Write Tuning 1", "Write Tuning 2", "Write Tuning 3" {
        # "Had to put a delay between CAN writes (mainly for the 3 tuning messages),\nor else the CAN would lock up on the micro."
        n124 = case shown="\"Write Tuning 2\"" w309 {
          tunnel: w310 -> [w317 w325 w331 w338]
          tunnel: [w316 w324 w330 w337] -> w311
          frame "Write Tuning 0", Default {
            n125 = call "CAN Floats to Message.vi"("Float_1"="ki", "Float_0"="kp") -> ("CAN Message"=w321:u8[])  [unwired: 9 in]
            n126 = Bundle By Name(cluster=w317, "CAN Msg"=w321, "ArbID"=u32 64) -> (w316:T2)
          }
          frame "Write Tuning 1" {
            n127 = call "CAN Floats to Message.vi"("Float_1"="ff", "Float_0"="pwm_rate") -> ("CAN Message"=w327:u8[])  [unwired: 9 in]
            n128 = Bundle By Name(cluster=w325, "CAN Msg"=w327, "ArbID"=u32 80) -> (w324:T2)
          }
          frame "Write Tuning 2" {
            n129 = call "CAN Floats to Message.vi"("Float_1"="boost", "Float_0"="hyst") -> ("CAN Message"=w333:u8[])  [unwired: 9 in]
            n130 = Bundle By Name(cluster=w331, "CAN Msg"=w333, "ArbID"=u32 82) -> (w330:T2)
          }
          frame "Write Tuning 3" {
            n131 = Build Array("pwm_min", "boost_delay") -> (w335:u8[])
            n132 = Bundle By Name(cluster=w338, "CAN Msg"=w335, "ArbID"=u32 85) -> (w337:T2)
          }
        }
        n133 = Wait (ms)(milliseconds to wait=u32 100) -> ()  [unwired: 1 out]
        n134 = Insert Into Array(array=w314, index=0, new element=string[] ["Write CAN"]) -> (w315:string[])
      }
      frame "Update Screen" {
        n135 = Unbundle By Name(w345) -> ("Cal Read 1"=→"Cal Read 1":sgl, "Cal Read 2"=→"Cal Read 2":sgl, "Cal Coeffs"=→"Cal Coeffs":sgl[], "Current Temp"=→"Temp (deg F)":sgl, "Temp (raw)"=→"Temp (raw)":sgl, "Parameter Received"=→"Parameters Received":bool, "Version"=→"Version":sgl)
        n136 = Unbundle By Name(w345) -> ("Current Temp"=w344:sgl, "Temp Setpoint (Live)"=w343:sgl, "PWM Command"=w342:sgl, "Integral"=w341:sgl)
        n137 = Build Array(w344, w343, w342, w341) -> (w347:sgl[])
        "Live Data" <- w347
        n138 = Array To Cluster(array=w347) -> (cluster=→"Tuning Chart":T1)
        n139 = Insert Into Array(array=w356, index=0, new element=string[] []) -> (w357:string[])
      }
      frame "Update Controls" {
        n140 = Unbundle By Name(w365) -> ("Cal Target 1"=w373:sgl, "Cal Target 2"=w372:sgl, "kp"=w371:sgl, "ki"=w370:sgl, "pwm_rate"=w369:sgl, "ff"=w364:sgl, "pwm_min"=w363:u8, "boost_delay"=w358:u8, "Temp Setpoint"=w368:sgl, "Output Enable"=w367:bool, "Output Enable Type"=w366:bool, "Alarm Diff"=w362:u8, "Alarm Enable"=w361:bool, "Mute Time (min)"=w360:u8, "Alarm State"=w359:bool)
        n141 = local write "boost_delay"(w358) -> ()
        n142 = local write "Cal Target 1"(w373) -> ()
        n143 = local write "Cal Target 2"(w372) -> ()
        n144 = local write "kp"(w371) -> ()
        n145 = local write "ki"(w370) -> ()
        n146 = local write "ff"(w364) -> ()
        n147 = local write "pwm_min"(w363) -> ()
        n148 = local write "Temp Setpoint"(w368) -> ()
        n149 = local write "Output Enable"(w367) -> ()
        n150 = local write "Output Enable Type"(w366) -> ()
        n151 = local write "Alarm Diff"(w362) -> ()
        n152 = local write "Alarm Enable"(w361) -> ()
        n153 = local write "Mute Time (min)"(w360) -> ()
        n154 = local write "Alarm State"(w359) -> ()
        n155 = local write "pwm_rate"(w369) -> ()
        n156 = Insert Into Array(array=w376, index=0, new element=string[] []) -> (w377:string[])
      }
      frame "Exit" {
        n157 = Unbundle By Name(w379) -> ("CAN Object"=w378:i32)
        n158 = call "closeneodevices.vi"("hObject"=w378) -> ()  [unwired: 2 in, 9 out]
        n159 = Insert Into Array(array=w382, index=0, new element=string[] []) -> (w383:string[])
      }
    }
  }
